vi "Configure Trigger (Slope).vi"(0 "VISA resource name":refnum<visa-resource-name>, 1 "Time Lower Limit (1E-6 s)":dbl=1e-06, 2 "Trigger Level Upper Limit (0)":dbl, 5 "Source (1: Channel 1)":i32(ring)=1 items=["Channel 1"=1, "Channel 2"=2, "Channel 3"=3, "Channel 4"=4], 7 "Trigger Condition (0: PGR)":i32(ring) items=["PGR", "PLES", "NGR", "NLES", "PGL", "NGL"], 9 "Time Upper Limit (2E-6 s)":dbl=2e-06, 11 "error in (no error)":errorcluster, 12 "Windows Type (0: TA)":i32(ring) items=["TA", "TB", "TAB"], 13 "Trigger Level Lower Limit (0)":dbl) -> (4 "VISA resource name out":refnum<visa-resource-name>, 15 "error out":errorcluster)   [LabVIEW 2015, in "ZhiYuan ZDS Series for TCP.lvlib"]
doc: "Configures the setting for slope trigger."
uses:
  ZhiYuan ZDS Series for TCP.lvlib
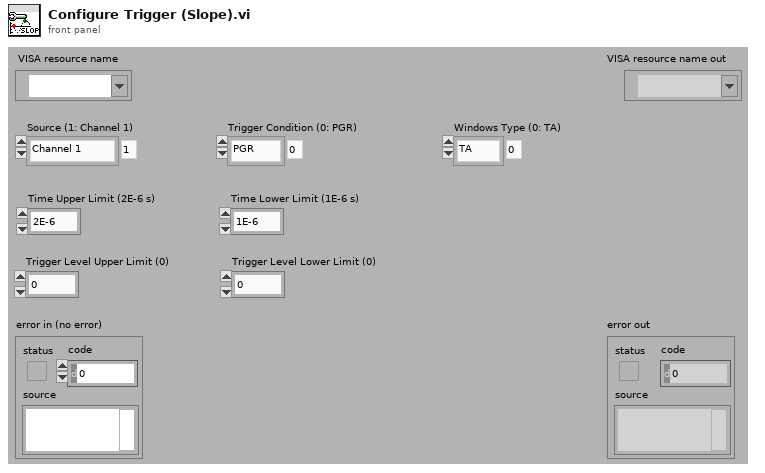
[diagram p1: front panel]
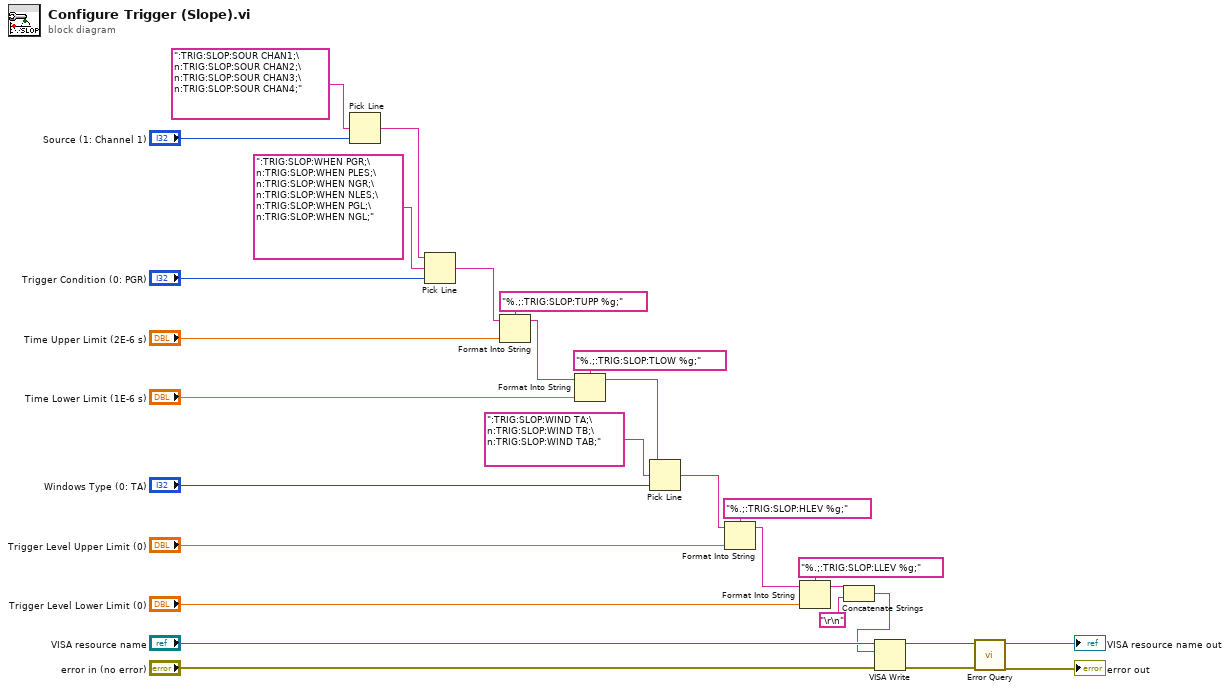
[diagram p0: block diagram]
diagram:
  n1 = Pick Line(multi-line string=":TRIG:SLOP:SOUR CHAN1;\n:TRIG:SLOP:SOUR CHAN2;\n:TRIG:SLOP:SOUR CHAN3;\n:TRIG:SLOP:SOUR CHAN4;", line index="Source (1: Channel 1)") -> (output string=w25:string)  [unwired: 1 in]
  n2 = Pick Line(string ("")=w25, multi-line string=":TRIG:SLOP:WHEN PGR;\n:TRIG:SLOP:WHEN PLES;\n:TRIG:SLOP:WHEN NGR;\n:TRIG:SLOP:WHEN NLES;\n:TRIG:SLOP:WHEN PGL;\n:TRIG:SLOP:WHEN NGL;", line index="Trigger Condition (0: PGR)") -> (output string=w24:string)
  n3 = Format Into String(format string="%.;:TRIG:SLOP:TUPP %g;", initial string=w24, "Time Upper Limit (2E-6 s)") -> (resulting string=w21:string)  [unwired: 1 in, 1 out]
  n4 = Format Into String(format string="%.;:TRIG:SLOP:TLOW %g;", initial string=w21, "Time Lower Limit (1E-6 s)") -> (resulting string=w16:string)  [unwired: 1 in, 1 out]
  n5 = Pick Line(string ("")=w16, multi-line string=":TRIG:SLOP:WIND TA;\n:TRIG:SLOP:WIND TB;\n:TRIG:SLOP:WIND TAB;", line index="Windows Type (0: TA)") -> (output string=w15:string)
  n6 = Format Into String(format string="%.;:TRIG:SLOP:HLEV %g;", initial string=w15, "Trigger Level Upper Limit (0)") -> (resulting string=w12:string)  [unwired: 1 in, 1 out]
  n7 = Format Into String(format string="%.;:TRIG:SLOP:LLEV %g;", initial string=w12, "Trigger Level Lower Limit (0)") -> (resulting string=w3:string)  [unwired: 1 in, 1 out]
  n8 = Concatenate Strings(w3, "\r\n") -> (w1:string)
  n9 = VISA Write(VISA resource name="VISA resource name", write buffer=w1, error in (no error)="error in (no error)") -> (VISA resource name out=w7:refnum<visa-resource-name>, error out=w6:errorcluster)  [unwired: 1 out]
  n10 = call "Error Query.vi"("error in (no error)"=w6, "VISA resource name"=w7) -> ("error out"=→"error out":errorcluster, "VISA resource name out"=→"VISA resource name out":refnum<visa-resource-name>)  [unwired: 6 in, 2 out]
